vi "FTW-CodeGen-FindGObject.vi"(0 "GObject to Traverse":refnum<vi>, 5 "Class Name":string, 11 "error in":errorcluster) -> (6 "GObject":refnum<vi>, 15 "error out":errorcluster)   [LabVIEW 2013, in "FTW-CodeGen.lvlib"]
uses:
  FTW-CodeGen.lvlib
  core/error/FTW-ERR-ThrowError.vi
  core/error/FTW-ERR-NoErrorConstant.vi
  core/error/FTW-ERR-CallChain.vi
  core/string/FTW-STR-ReplaceWhitespace.vi
panel:
  # "Inputs"
  # "Outputs"
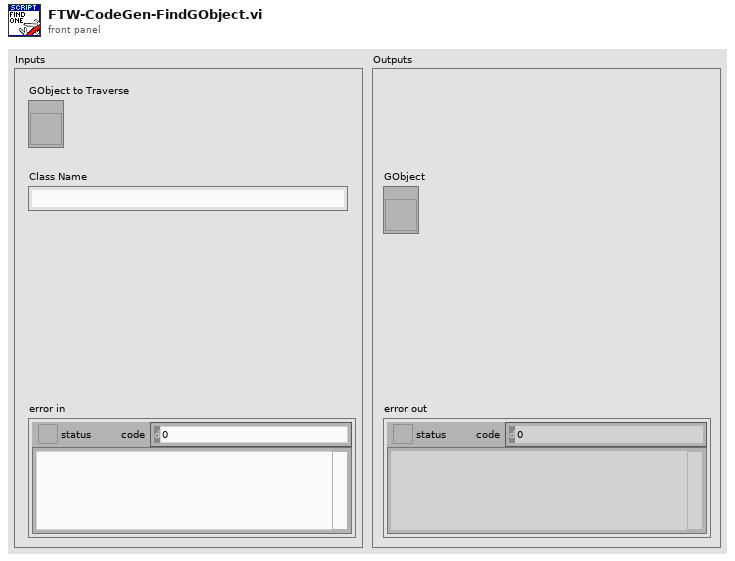
[diagram p1: front panel]
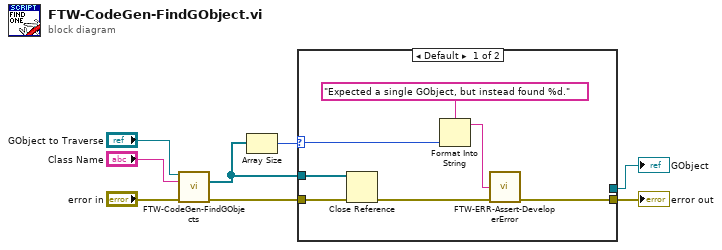
[diagram p0: block diagram]
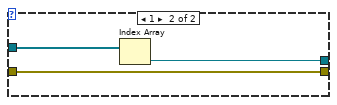
[diagram p2: hidden frame]
diagram:
  n1 = call "FTW-CodeGen-FindGObjects.vi"("GObject to Traverse"="GObject to Traverse", "Class Name"="Class Name", "error in"="error in") -> ("GObject Instances"=w2:refnum<vi>[], "error out"=w3:errorcluster)  [unwired: 11 in]
  n2 = Array Size(array=w2) -> (size(s)=w5:i32)
  n3 = case shown="Default" w5 {
    selector: w5 -> [w13 _]
    tunnel: [w15 w18] -> w4
    tunnel: w3 -> [w10 w18]
    tunnel: w2 -> [w11 w17]
    tunnel: [_ w16] -> w1
    frame Default {
      n4 = Close Reference(reference=w11, error in (no error)=w10) -> (error out=w9:errorcluster)
      n5 = Format Into String(format string="Expected a single GObject, but instead found %d." ("Reason this error should never happen"), w13) -> (resulting string=w12:string)  [unwired: 2 in, 1 out]
      n6 = call "FTW-ERR-Assert-DeveloperError.vi"("Reason this error should never happen"=w12, "error in"=w9) -> ("error out"=w15:errorcluster)  [unwired: 13 in]
    }
    frame 1 {
      n7 = Index Array(array=w17) -> (element=w16:refnum<vi>)  [unwired: 1 in]
    }
  }
  "error out" <- w4
  "GObject" <- w1
